vi "Get Parameter Name.vi"(8 "error in":errorcluster, 11 "parameter ref":T1 format="%.0x") -> (0 "error out":errorcluster, 2 "name":string, 3 "parameter ref out":T1 format="%.0x")   [LabVIEW 2020, in "AIM ARINC 429 Scripting.lvlib"]
uses:
  <vilib>/NI VeriStand/Custom Device API/Custom Device Item Ref.ctl
  AIM/AIM ARINC 429 Scripting.lvlib
  <vilib>/NI VeriStand/Custom Device API/Custom Device API.lvlib
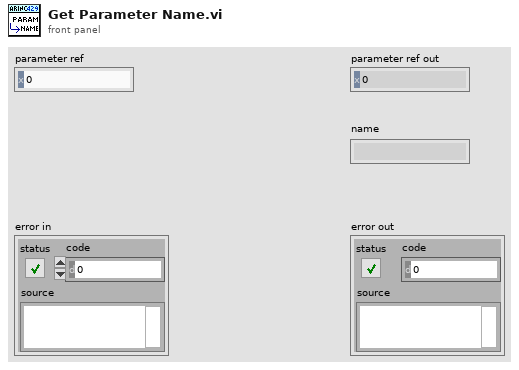
[diagram p1: front panel]
types:
  T1 = typedef "Custom Device API.lvlib/Custom Device Item Ref.ctl" = u64
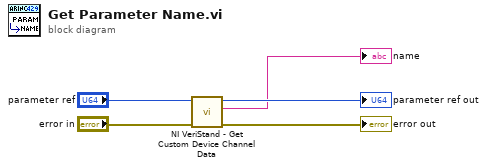
[diagram p0: block diagram]
diagram:
  n1 = call <vilib>:"NI VeriStand - Get Custom Device Channel Data.vi"("error in (no error)"="error in", "Channel Ref in"="parameter ref") -> ("error out"=→"error out":errorcluster, "Channel Name"=→"name":string, "Channel Ref out"=→"parameter ref out":T1)  [unwired: 4 in, 3 out]
